vi "Lid Lock (SLB).vi"(0 "GEA2 Reference In":refnum<k24>, 2 "Standalone?":bool, 5 "GEA Inputs":T1={"Source"=228, "Destination"=35} {"Destination" format="%.0x"; "Source" format="%.0x"}, 7 "Action":enum16{"Unlock", "Lock"}(ring), 11 "Error In":errorcluster) -> (4 "GEA2 Reference Out":refnum<k24>, 6 "Pass/Fail?":bool, 8 "Report Text":string, 15 "Error Out":errorcluster)   [LabVIEW 2016, in "TL27.lvlib"]
uses:
  Projects/TL27.lvlib
  C:/Automation/DLLs/PC Dot Net/GeaCommunication.dll
  Common/LabVIEW GEA2 Toolkit/LabVIEW_GEA2_Toolkit.lvlibp/type defs/Source_Destination.ctl
  Common/LabVIEW GEA2 Toolkit/LabVIEW_GEA2_Toolkit.lvlibp/type defs/ERD Read Data In.ctl
  Common/LabVIEW GEA2 Toolkit/LabVIEW_GEA2_Toolkit.lvlibp/type defs/Data Type.ctl
  Common/LabVIEW GEA2 Toolkit/LabVIEW_GEA2_Toolkit.lvlibp/type defs/ERD Write Data In.ctl
  <vilib>/DAQmx/write.llb/DAQmx Write (Digital 1D Wfm NChan NSamp).vi
  <vilib>/DAQmx/create/channels.llb/DAQmx Create Channel (DO-Digital Output).vi
  <vilib>/DAQmx/configure/timing.llb/DAQmx Timing (Sample Clock).vi
  <vilib>/DAQmx/configure/trigger.llb/DAQmx Start Trigger (Digital Edge).vi
  <vilib>/Waveform/DTblOps.llb/DTbl Boolean Array to Digital.vi
  <vilib>/Waveform/DWDTOps.llb/DWDT Uncompress Digital.vi
  <vilib>/DAQmx/miscellaneous.llb/DAQmx Fill In Error Info.vi
  Common/LabVIEW GEA2 Toolkit/LabVIEW_GEA2_Toolkit.lvlibp
  <resource>/objmgr/daqmx.rc
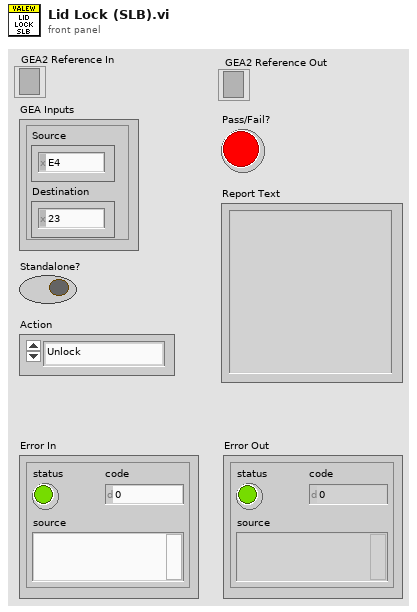
[diagram p1: front panel]
types:
  T1 = typedef "LabVIEW_GEA2_Toolkit.lvlibp/Source_Destination.ctl" = cluster{"Source":u8, "Destination":u8}
  T2 = typedef "LabVIEW_GEA2_Toolkit.lvlibp/ERD Read Data In.ctl" = cluster{"ERD Number":u16, "Data Type":T3}
  T3 = typedef "LabVIEW_GEA2_Toolkit.lvlibp/Data Type.ctl" = enum16{"string", "boolean", "uint8_t", "uint16_t", "uint32_t", "uint64_t", "int8_t", "int16_t", "int32_t", "int64_t"}
  T4 = typedef "LabVIEW_GEA2_Toolkit.lvlibp/ERD Write Data In.ctl" = cluster{"ERD Number":u16, "Data Type":T3, "Data":string}
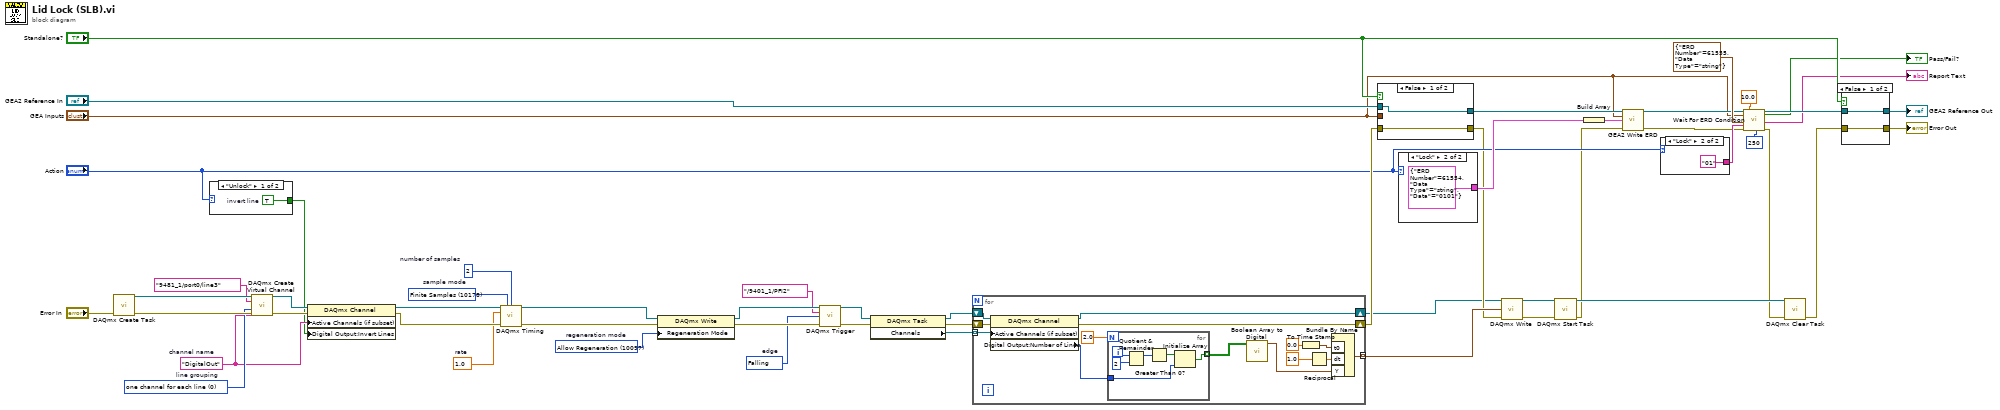
[diagram p0: block diagram]
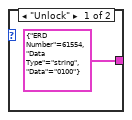
[diagram p2: hidden frame]
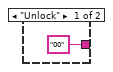
[diagram p3: hidden frame]
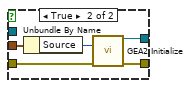
[diagram p4: hidden frame]
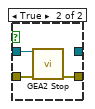
[diagram p5: hidden frame]
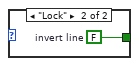
[diagram p6: hidden frame]
diagram:
  w31 = 10171 items=["Rising"=10280, "Falling"=10171]  # edge
  w33 = 10097 items=["Allow Regeneration"=10097, "Do Not Allow Regeneration"=10158]  # regeneration mode
  w36 = 10178 items=["Finite Samples"=10178, "Continuous Samples"=10123, "Hardware Timed Single Point"=12522]  # sample mode
  w37 = 2  # number of samples
  w38 = 1.0  # rate
  w45 = 0 items=["one channel for each line", "one channel for all lines"]  # line grouping
  w41 = "DigitalOut"  # channel name
  n1 = call <vilib>:"DAQmx Create Task.vi"("error in"="Error In") -> ("task out"=w46:refnum<k21>, "error out"=w47:errorcluster)  [unwired: 13 in]
  n2 = case shown="\"Unlock\"" "Action" {
    tunnel: [w55 w56] -> w19
    frame "Unlock" {
      w55 = TRUE  # invert line
    }
    frame "Lock" {
      w56 = FALSE  # invert line
    }
  }
  n3 = call-poly <vilib>:"DAQmx Create Virtual Channel.vi"("task in"=w46, "lines"=tag "9481_1/port0/line3", "name to assign"=w41, "line grouping"=w45, "error in"=w47) -> ("task out"=w44:refnum<k21>, "error out"=w43:errorcluster)  [unwired: 9 in]
  n4 = property class="DAQmx Channel"(reference=w44, error in=w43, "Active Channels (if subset)"=w41, "Digital Output:Invert Lines"=w19) -> (reference out=w39:refnum<k21>, error out=w42:errorcluster)
  n5 = call-poly <vilib>:"DAQmx Timing.vi"("task/channels in"=w39, "sample mode"=w36, "samples per channel"=w37, "rate"=w38, "error in"=w42) -> ("task out"=w35:refnum<k21>, "error out"=w40:errorcluster)  [unwired: 9 in]
  n6 = property class="DAQmx Write"(reference=w35, error in=w40, "Regeneration Mode"=w33) -> (reference out=w32:refnum<k21>, error out=w34:errorcluster)
  n7 = call-poly <vilib>:"DAQmx Trigger.vi"("task/channels in"=w32, "source"=tag "/9401_1/PFI2", "edge"=w31, "error in"=w34) -> ("task out"=w29:refnum<k21>, "error out"=w28:errorcluster)  [unwired: 10 in]
  n8 = property class="DAQmx Task"(reference=w29, error in=w28) -> (reference out=w27:refnum<k21>, error out=w18:errorcluster, "Channels"=w30:refnum<k21>[])
  n9 = for {
    tunnel: [w66] -> w26 mode=indexing
    tunnel: w30 -> [w64] mode=indexing
    shift-right: [w58] -> w17
    shift-left: w18 -> [w59]
    shift-right: [w57] -> w3
    shift-left: w27 -> [w62]
    n10 = property class="DAQmx Channel"(reference=w62, error in=w59, "Active Channels (if subset)"=w64) -> (reference out=w57:refnum<k21>, error out=w58:errorcluster, "Digital Output:Number of Lines"=w63:u32)
    n11 = for {
      N: 2.0 ("number of samples") -> [_]
      tunnel: [w71] -> w65 mode=indexing
      tunnel: w63 -> [w72]
      i -> [w76]
      n12 = Quotient & Remainder(x=w76, y=2) -> (x-y*floor(x/y)=w74:i32)  [unwired: 1 out]
      n13 = Greater Than 0?(x=w74) -> (x > 0?=w73:bool)
      n14 = Initialize Array(w73, w72) -> (w71:bool[])
    }
    n15 = call-poly <vilib>:"Boolean Array to Digital.vi"("boolean array"=w65) -> ("digital data"=w68:digitaldata)  [unwired: 3 in, 7 out]
    n16 = To Time Stamp(1:0.0) -> (0:w69:timestamp)
    n17 = Reciprocal(x=1.0 ("update rate")) -> (1/x=w67:dbl)
    n18 = Bundle By Name("t0"=w69, "dt"=w67, "Y"=w68) -> (w66:digitalwaveform)  [unwired: 1 out]
  }
  n19 = case shown="False" "Standalone?" {
    tunnel: w17 -> [w77 w83]
    tunnel: [w77 w82] -> w6
    tunnel: "GEA2 Reference In" -> [w78 _]
    tunnel: [w78 w81] -> w50
    tunnel: "GEA Inputs" -> [_ w79]
    frame False {
    }
    frame True {
      n20 = Unbundle By Name(w79) -> ("Source"=w80:u8)
      n21 = call "GEA2 Initialize.vi"("Source Address"=w80, "error in"=w83) -> ("GEA2 Reference Out"=w81:refnum<k24>, "error out"=w82:errorcluster)  [unwired: 11 in, 1 out]
    }
  }
  n22 = case shown="\"Lock\"" "Action" {
    tunnel: [T4 {"ERD Number"=61554, "Data Type"=enum."string", "Data"="0100"} ("ERD Write Data In") T4 {"ERD Number"=61554, "Data Type"=enum."string", "Data"="0101"} ("ERD Write Data In")] -> w13
    frame "Unlock" {
    }
    frame "Lock" {
    }
  }
  n23 = call-poly <vilib>:"DAQmx Write.vi"("task/channels in"=w3, "data"=w26, "error in"=w6) -> ("task out"=w49:refnum<k21>, "error out"=w48:errorcluster)  [unwired: 10 in, 1 out]
  n24 = call <vilib>:"DAQmx Start Task.vi"("task/channels in"=w49, "error in"=w48) -> ("task out"=w9:refnum<k21>, "error out"=w5:errorcluster)  [unwired: 12 in]
  n25 = Build Array(w13) -> (w54:T4[])
  n26 = call "GEA2 Write ERD.vi"("GEA2 Reference In"=w50, "GEA Inputs"="GEA Inputs", "Write ERD List"=w54, "Error In"=w5) -> ("GEA2 Reference Out"=w23:refnum<k24>, "Error Out"=w4:errorcluster)  [unwired: 9 in, 1 out]
  n27 = case shown="\"Lock\"" "Action" {
    tunnel: ["00" ("y") "01" ("y")] -> w24
    frame "Unlock" {
    }
    frame "Lock" {
    }
  }
  n28 = call "Wait For ERD Condition.vi"("GEA2 Reference In"=w23, "GEA Inputs"="GEA Inputs", "ERD Read Data"=T2 {"ERD Number"=61555, "Data Type"=enum."string"} ("ERD Read Data In"), "Expected Low"=w24, "Error In"=w4, "Timeout (s)"=10.0, "Loop Rate (ms)"=u32 250) -> ("GEA2 Reference Out"=w21:refnum<k24>, "Pass/Fail?"=→"Pass/Fail?":bool, "Report Text"=→"Report Text":string, "Error Out"=w8:errorcluster)  [unwired: 8 in, 1 out]
  n29 = call <vilib>:"DAQmx Clear Task.vi"("task in"=w9, "error in"=w8) -> ("error out"=w7:errorcluster)  [unwired: 13 in]
  n30 = case shown="False" "Standalone?" {
    tunnel: w21 -> [w89 w92]
    tunnel: w7 -> [w88 w91]
    tunnel: [w88 w90] -> w10
    tunnel: [w89 _] -> w51
    frame False {
    }
    frame True {
      n31 = call "GEA2 Stop.vi"("GEA2 Reference In"=w92, "Error In"=w91) -> ("Error Out"=w90:errorcluster)  [unwired: 13 in]
    }
  }
  "GEA2 Reference Out" <- w51
  "Error Out" <- w10
